vi "Configure Noise.vi"(6 "Units (0: Volt)":i32(ring) items=["Volt", "Unit Amplitude"], 7 "Enable Noise Measurement (F: Disable)":bool, 8 "error in (no error)":errorcluster, 9 "Measurement Location (50)":dbl=50.0, 10 "Filter Type (1: Wide)":i32(ring)=1 items=["Narrow", "Wide"], 11 "VISA resource name":refnum<visa-resource-name>) -> (0 "error out":errorcluster, 3 "VISA resource name out":refnum<visa-resource-name>)   [LabVIEW 2013, in "Agilent 90000 Series.lvlib"]
doc: "Configures settings of noise measurement.\n\n<B>Note:</B>\nThis VI is only available when the EZJIT Complete software is installed."
uses:
  Agilent 90000 Series.lvlib
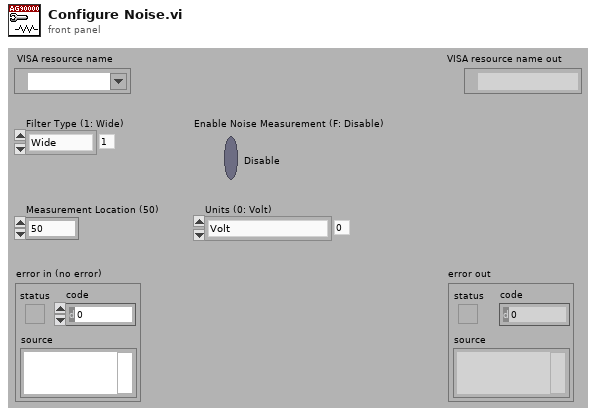
[diagram p1: front panel]
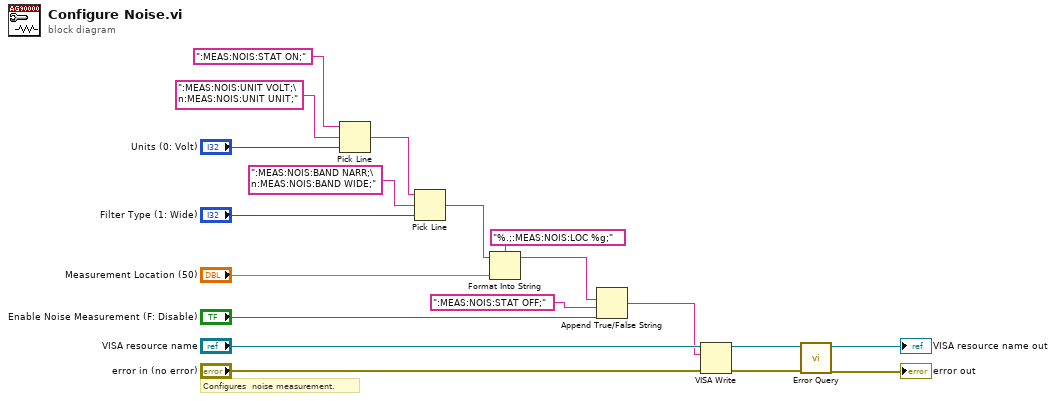
[diagram p0: block diagram]
diagram:
  # "Configures  noise measurement."
  n1 = Pick Line(string ("")=":MEAS:NOIS:STAT ON;", multi-line string=":MEAS:NOIS:UNIT VOLT;\n:MEAS:NOIS:UNIT UNIT;", line index="Units (0: Volt)") -> (output string=w13:string)
  n2 = Pick Line(string ("")=w13, multi-line string=":MEAS:NOIS:BAND NARR;\n:MEAS:NOIS:BAND WIDE;", line index="Filter Type (1: Wide)") -> (output string=w12:string)
  n3 = Format Into String(format string="%.;:MEAS:NOIS:LOC %g;", initial string=w12, "Measurement Location (50)") -> (resulting string=w2:string)  [unwired: 1 in, 1 out]
  n4 = Append True/False String(1:"Enable Noise Measurement (F: Disable)", 2:":MEAS:NOIS:STAT OFF;", 3:w2) -> (0:w1:string)  [unwired: 1 out]
  n5 = VISA Write(VISA resource name="VISA resource name", write buffer=w1, error in (no error)="error in (no error)") -> (VISA resource name out=w7:refnum<visa-resource-name>, error out=w6:errorcluster)  [unwired: 1 out]
  n6 = call "Error Query.vi"("error in (no error)"=w6, "VISA resource name"=w7) -> ("error out"=→"error out":errorcluster, "VISA resource name out"=→"VISA resource name out":refnum<visa-resource-name>)  [unwired: 8 out]
